vi "client.vi"() -> ()   [LabVIEW 2017]
uses:
  9d727d11-b689-4871-8819-2053d65de9d0.vi
  893ad8d0-d08f-485b-b6ee-436a327f275c.vi
  <vilib>/dlg_ctls.llb/Space Constant.vi
  <vilib>/NI/JSON Support for LabVIEW/JSON Value/New JSON Value.vi
  <vilib>/NI/JSON Support for LabVIEW/JSON Value/New JSON Value/New JSON ({}).vi
  <vilib>/Utility/Data Type/Get Type Information.vi
  <vilib>/Utility/Data Type/Get Array Information.vi
  <vilib>/NI/JSON Support for LabVIEW/JSON Value/Object/Insert Value.vi
  <vilib>/NI/JSON Support for LabVIEW/JSON Value/Object/Insert Value/Insert Value (String).vi
  <vilib>/NI/JSON Support for LabVIEW/JSON Value/Object/Insert Value/Insert Value (Numeric).vi
  <vilib>/NI/NI JSONRPC Server Framework/Classes/Client/Format Client Request.vi
  <vilib>/NI/NI JSONRPC Server Framework/Classes/Client/Format Client Request (Auto-Increment).vi
  <vilib>/httpClient/POST.vi
  <vilib>/httpClient/POSTBuffer.vi
  <vilib>/NI/NI JSONRPC Server Framework/Classes/Client/Parse Response for Result or Error.vi
  <vilib>/NI/JSON Support for LabVIEW/JSON Value/Object/Get Value.vi
  <vilib>/NI/JSON Support for LabVIEW/JSON Value/Object/Get Value/Get Value (Value).vi
  <vilib>/NI/JSON Support for LabVIEW/JSON Value/Helper Methods/To String.vi
  client/DCAF_JSON_RPC_client.lvlib
panel:
  in  "stop":bool
  out "DBL0Read":dbl
  out "error out 4":errorcluster
  in  "DBL0Write":dbl format="%#_13g"
  out "error out":errorcluster
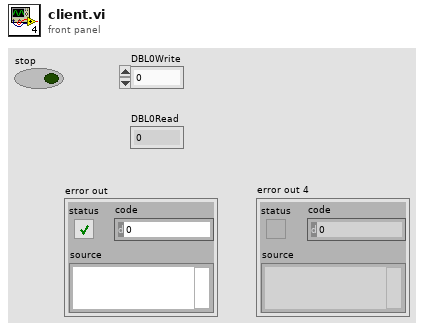
[diagram p1: front panel]
types:
  T1 = typedef "DCAF_JSON_RPC_client.lvlib/handle.ctl" = cluster{"uri":string, " clientRef in":T2}
  T2 = typedef "LabVIEWHTTPClient.lvlib/ClientHandle.ctl" = refnum<k1>
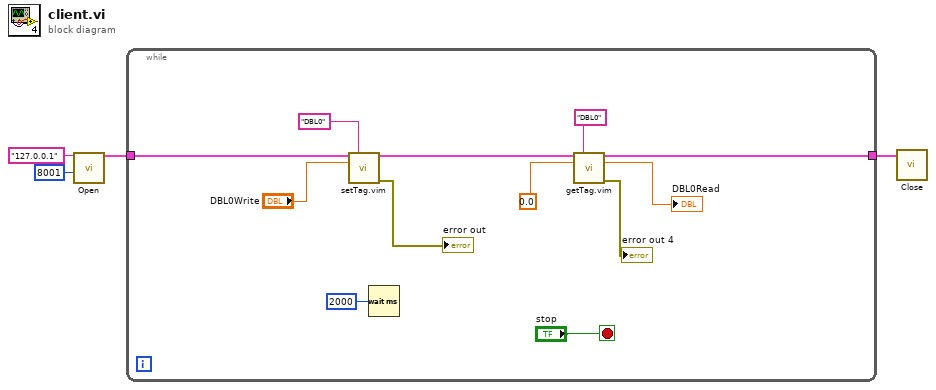
[diagram p0: block diagram]
diagram:
  n1 = call "Open.vi"("ip"="127.0.0.1", "port"=u16 8001) -> ("handle out"=w1:T1)  [unwired: 12 in, 1 out]
  n2 = while {
    tunnel: w1 -> [w16]
    tunnel: [w13] -> w2
    stop <- "stop" stop-if-true
    n3 = call "setTag.vim"("handle in"=w16, "tagname"="DBL0", "tagdata"="DBL0Write") -> ("handle out"=w8:T1, "error out"=→"error out":errorcluster)  [unwired: 9 in, 2 out]
    n4 = Wait (ms)(milliseconds to wait=u32 2000) -> ()  [unwired: 1 out]
    n5 = call "getTag.vim"("handle in"=w8, "tagname"="DBL0", "default"=0.0 ("Numeric")) -> ("handle out"=w13:T1, "value"=→"DBL0Read":dbl, "error out"=→"error out 4":errorcluster)  [unwired: 8 in, 2 out]
  }
  n6 = call "Close.vi"("handle in"=w2) -> ()  [unwired: 14 in, 1 out]
